vi "EX 10.vi"() -> ()   [LabVIEW 2018]
panel:
  in  "moyenne visée":dbl
  out "6 ieme note":dbl
  out "Tableau":dbl[](array[numeric])
  in  "stop":bool
  in  "Moyenne":dbl
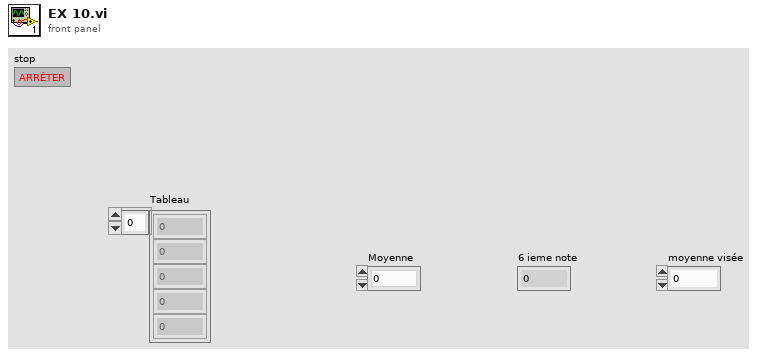
[diagram p1: front panel]
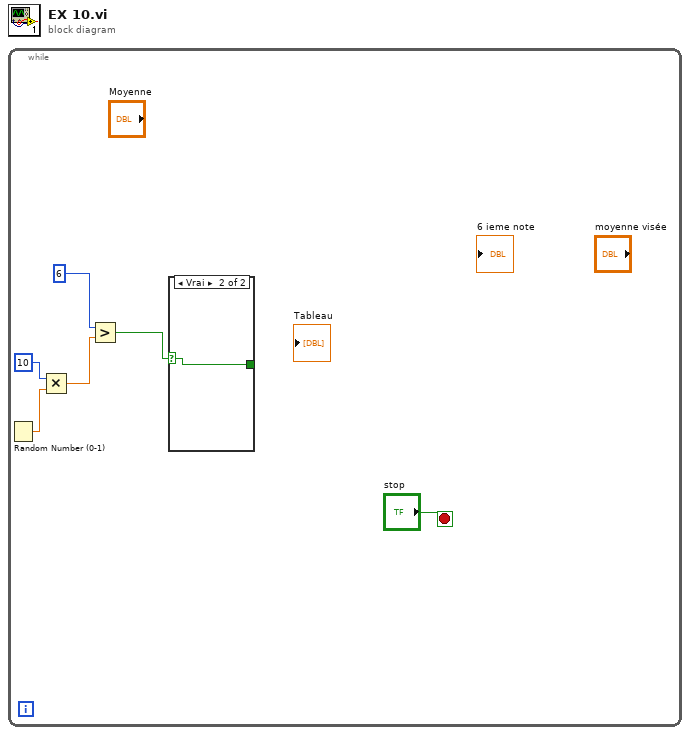
[diagram p0: block diagram]
diagram:
  n1 = while {
    stop <- "stop" stop-if-true
    n2 = Random Number (0-1) ("Nombre aléatoire (0.3-0.6)")() -> (number: 0 to 1=w5:dbl)
    n3 = Multiply(x=10, y=w5) -> (x*y=w3:dbl)
    n4 = Greater?(x=6, y=w3) -> (0:w1:bool)
    n5 = case shown="Vrai" w1 {
      selector: w1 -> [_ w7]
      tunnel: [_ w7] -> _
      frame False {
      }
      frame True {
      }
    }
  }
